vi "Platform Names.vi"(8 "error in (no error)":errorcluster, 11 "TargetPluginManager in":refnum<class "PlatformPluginManager.lvclass">) -> (0 "error out":errorcluster, 2 "Platforms":string[](array[string]), 3 "TargetPluginManager out":refnum<class "PlatformPluginManager.lvclass">)   [LabVIEW 2020, in "PicoG-Core.lvlib" / "PlatformPluginManager.lvclass"]
uses:
  PlatformPluginManager.lvclass
  PlatformPluginManager.lvclass/PlatformPluginManager.ctl
  DeployPlatform/DeployPlatform.lvclass
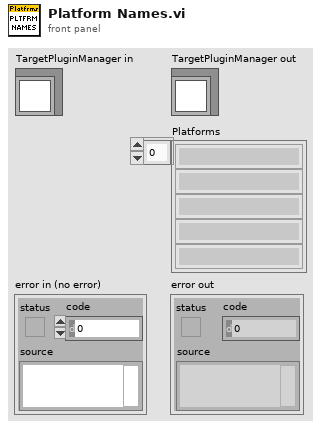
[diagram p1: front panel]
types:
  T1 = typedef "PicoG-Core.lvlib/PlatformPluginManager.lvclass/Ref Data.ctl" = cluster{"Platforms":refnum<class "DeployPlatform.lvclass">[], "Last Platform":refnum<class "DeployPlatform.lvclass">, "Last Resource":refnum<class "DeployResource.lvclass">}
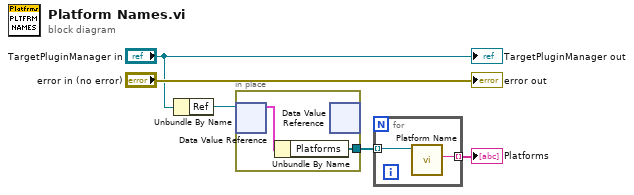
[diagram p0: block diagram]
diagram:
  n1 = Unbundle By Name("TargetPluginManager in") -> ("Ref"=w4:refnum<data-value>)
  n2 = in-place {
    in-place-border: [w6] -> w2
    n3 = in-place-dvr #1(w4) -> (w7:T1)  [unwired: 1 out]
    n4 = Unbundle By Name(w7) -> ("Platforms"=w6:refnum<class "DeployPlatform.lvclass">[])
    n5 = in-place-dvr #1() -> ()  [unwired: 1 in, 2 out]
  }
  n6 = for {
    tunnel: w2 -> [w9] mode=indexing
    tunnel: [w8] -> w1 mode=indexing
    n7 = call-dynamic "Platform Name.vi"("DeployTarget in"=w9) -> ("Platform Name"=w8:string)  [unwired: 8 in, 2 out]
  }
  "Platforms" <- w1
  "error out" <- "error in (no error)"
  "TargetPluginManager out" <- "TargetPluginManager in"
